vi "Miniquads.Close.vi"(0 "i ref in":refnum<vi>, 3 "ms timeout (10000)":i32=10000, 5 "error in (no error)":errorcluster) -> (14 "i ref out":refnum<vi>, 17 "timed out":bool, 19 "error out":errorcluster)   [LabVIEW 2014, in "Miniquads.lvlib"]
doc: "This vi unloads the previously created objects."
uses:
  Miniquads.lvlib
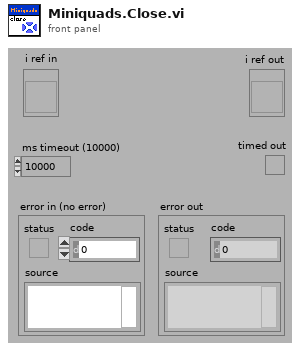
[diagram p1: front panel]
types:
  T1 = typedef "Miniquads.lvlib/Miniquads.i attribute.ctl" = cluster{"ObjectsInitialized":bool, "ObjectsLoaded":string[], "nomValues":T2, "actValues":T2}
  T2 = typedef "Miniquads.lvlib/Miniquads.voltages.ctl" = cluster{"FocusVoltage":dbl, "HorizontalVoltage":dbl, "VerticalVoltage":dbl, "serviceIDs":cluster{"FocusVoltageID":i32, "HorizontalVoltageID":i32, "VerticalVoltageID":i32}}
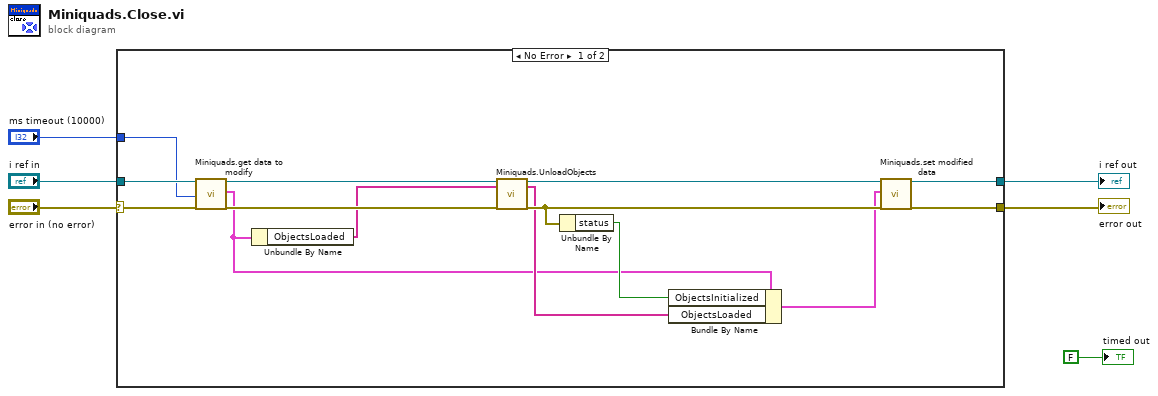
[diagram p0: block diagram]
diagram:
  n1 = case shown="No Error" "error in (no error)" {
    selector: "error in (no error)" -> [w19 w21]
    tunnel: "i ref in" -> [w20 w22]
    tunnel: [w16 w22] -> w5
    tunnel: [w15 w21] -> w3
    tunnel: "ms timeout (10000)" -> [w18 _]
    frame No Error {
      n2 = call "Miniquads.get data to modify.vi"("i ref in"=w20, "ms timeout (10000)"=w18, "error in (no error)"=w19) -> ("i ref out"=w12:refnum<vi>, "i attribute"=w8:T1, "error out"=w11:errorcluster)  [unwired: 13 in, 1 out]
      n3 = Unbundle By Name(w8) -> ("ObjectsLoaded"=w10:string[])
      n4 = call "Miniquads.UnloadObjects.vi"("i ref in"=w12, "ObjectsLoaded in"=w10, "error in (no error)"=w11) -> ("i ref out"=w17:refnum<vi>, "ObjectsLoaded out"=w13:string[], "error out"=w14:errorcluster)  [unwired: 14 in]
      n5 = Unbundle By Name(w14) -> ("status"=w9:bool)
      n6 = Bundle By Name(cluster=w8, "ObjectsInitialized"=w9, "ObjectsLoaded"=w13) -> (w7:T1)
      n7 = call "Miniquads.set modified data.vi"("i ref in"=w17, "i attribute"=w7, "error in (no error)"=w14) -> ("i ref out"=w16:refnum<vi>, "error out"=w15:errorcluster)  [unwired: 15 in]
    }
    frame Error {
    }
  }
  "error out" <- w3
  "i ref out" <- w5
  "timed out" <- FALSE ("timed out")
